vi "set_version_number.vi"(8 "error in (no error)":errorcluster, 11 "HelioUpdateMH100803 in":refnum<class "HelioUpdateMH100803.lvclass">) -> (0 "error out":errorcluster, 3 "HelioUpdateMH100803 out":refnum<class "HelioUpdateMH100803.lvclass">)   [LabVIEW 2010, in "HelioUpdateMH100803.lvclass"]
uses:
  HelioUpdateMH100803.lvclass
panel:
  in  "revision":u8 max=99
  in  "minor":u8 max=99
  in  "mayor":u8 max=99
  # "Set new version number"
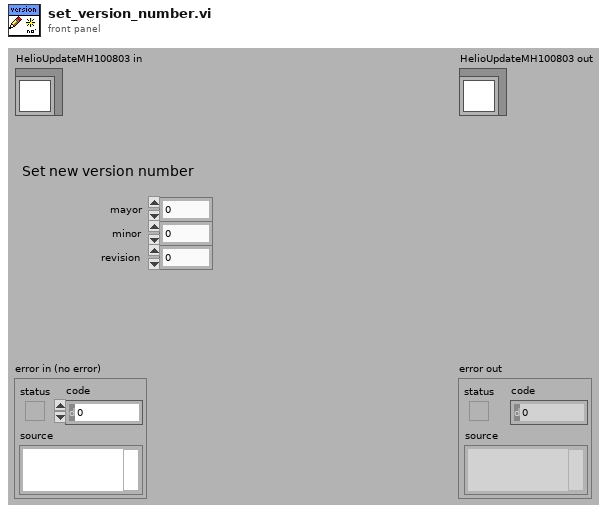
[diagram p1: front panel]
types:
  T1 = enum16{"open", "replace", "create", "open or create", "replace or create", "replace or create with confirmation"}
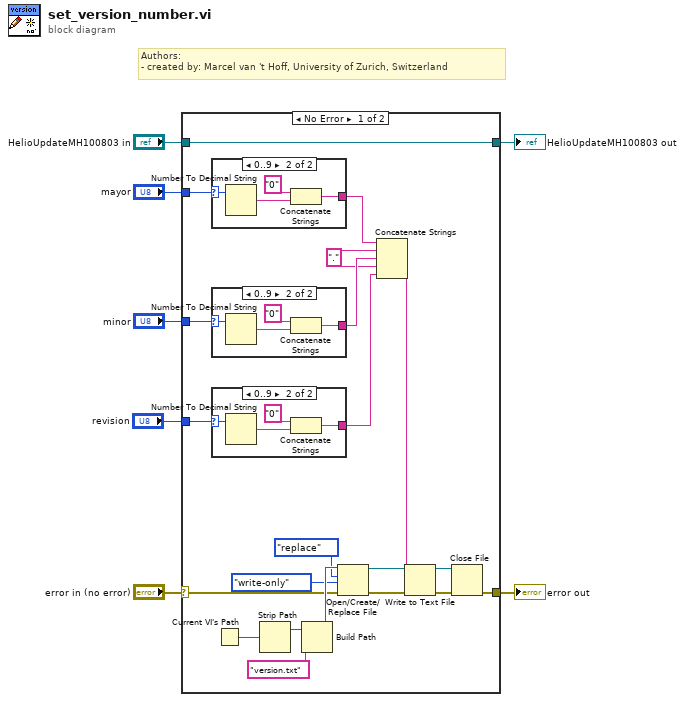
[diagram p0: block diagram]
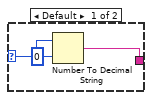
[diagram p2: hidden frame]
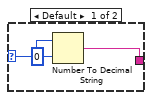
[diagram p3: hidden frame]
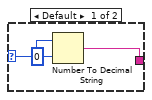
[diagram p4: hidden frame]
diagram:
  # "Authors: \n- created by: Marcel van 't Hoff, University of Zurich, Switzerland"
  n1 = case shown="No Error" "error in (no error)" {
    selector: "error in (no error)" -> [w23 w51]
    tunnel: [w22 w51] -> w6
    tunnel: [w28 w50] -> w4
    tunnel: "HelioUpdateMH100803 in" -> [w28 w50]
    tunnel: "mayor" -> [w14 _]
    tunnel: "minor" -> [w12 _]
    tunnel: "revision" -> [w10 _]
    frame No Error {
      w9 = "." ("string")
      n2 = case shown="0..9" w14 {
        selector: w14 -> [w45 w49]
        tunnel: [w44 w46] -> w13
        frame Default {
          n3 = Number To Decimal String(number=w45, width (-)=i16 0) -> (decimal integer string=w44:string)
        }
        frame 0..9 {
          n4 = Number To Decimal String(number=w49) -> (decimal integer string=w47:string)  [unwired: 1 in]
          n5 = Concatenate Strings("0" ("string"), w47) -> (w46:string)
        }
      }
      n6 = case shown="0..9" w12 {
        selector: w12 -> [w38 w42]
        tunnel: [w37 w39] -> w11
        frame Default {
          n7 = Number To Decimal String(number=w38, width (-)=i16 0) -> (decimal integer string=w37:string)
        }
        frame 0..9 {
          n8 = Number To Decimal String(number=w42) -> (decimal integer string=w40:string)  [unwired: 1 in]
          n9 = Concatenate Strings("0" ("string"), w40) -> (w39:string)
        }
      }
      n10 = case shown="0..9" w10 {
        selector: w10 -> [w31 w35]
        tunnel: [w30 w32] -> w8
        frame Default {
          n11 = Number To Decimal String(number=w31, width (-)=i16 0) -> (decimal integer string=w30:string)
        }
        frame 0..9 {
          n12 = Number To Decimal String(number=w35) -> (decimal integer string=w33:string)  [unwired: 1 in]
          n13 = Concatenate Strings("0" ("string"), w33) -> (w32:string)
        }
      }
      n14 = Current VI's Path() -> (path=w25:path)
      n15 = Strip Path(path=w25) -> (stripped path=w27:path)  [unwired: 1 out]
      n16 = Build Path(base path=w27, name or relative path="version.txt") -> (appended path=w24:path)
      n17 = Open/Create/Replace File(file path (use dialog)=w24, error in=w23, operation (0:open)=T1."replace", access (0:read/write)=enum16{"read/write", "read-only", "write-only"}."write-only") -> (refnum out=w17:refnum<file>, error out=w19:errorcluster)  [unwired: 2 in, 1 out]
      n18 = Concatenate Strings(w13, w9, w11, w9, w8) -> (w15:string)
      n19 = Write to Text File(file (use dialog)=w17, text=w15, error in=w19) -> (refnum out=w16:refnum<file>, error out=w18:errorcluster)  [unwired: 1 in, 1 out]
      n20 = Close File(refnum=w16, error in=w18) -> (error out=w22:errorcluster)  [unwired: 1 out]
    }
    frame Error {
    }
  }
  "error out" <- w6
  "HelioUpdateMH100803 out" <- w4
